vi "Position Error Dialog.vi"(10 "Err Dialog Ref":refnum<vi>, 11 "DAQMan Ref":refnum<vi>) -> (2 "Dialog Ref Out":refnum<vi>)   [LabVIEW 2012, in "Configuration Grandmaster.lvlib" / "FP Controls.lvclass"]
uses:
  FP Controls.lvclass
  <vilib>/Utility/miscctls.llb/LVRectTypeDef.ctl
panel:
  out "output cluster":T1
  out "Front Panel Window:Window Bounds":T1
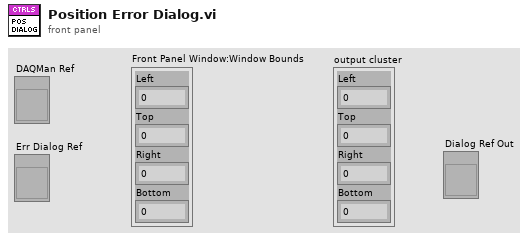
[diagram p1: front panel]
types:
  T1 = typedef "LVRectTypeDef.ctl" = cluster{"Left":i16, "Top":i16, "Right":i16, "Bottom":i16}
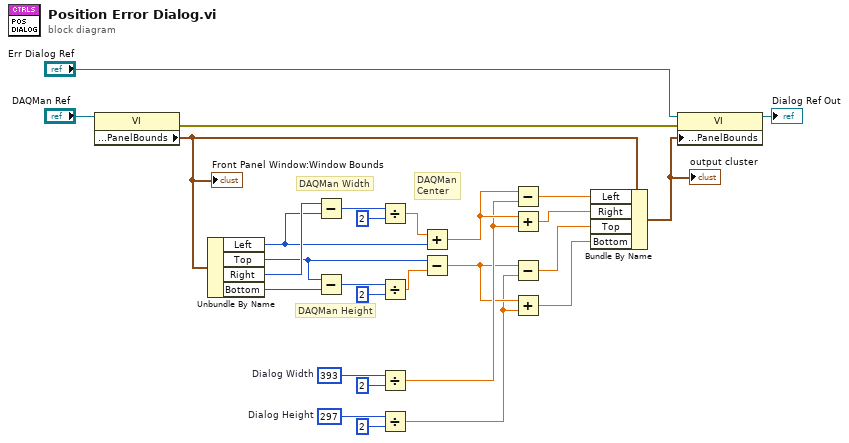
[diagram p0: block diagram]
diagram:
  w16 = i16 297  # Dialog Height
  w18 = i16 393  # Dialog Width
  # "DAQMan\nCenter"
  # "DAQMan Height"
  # "DAQMan Width"
  n1 = property class="VI"(reference="DAQMan Ref") -> (error out=w28:errorcluster, "Front Panel.PanelBounds"=w11:T1)  [unwired: 1 in, 1 out]
  "Front Panel Window:Window Bounds" <- w11
  n2 = Unbundle By Name(w11) -> ("Left"=w15:i16, "Top"=w13:i16, "Right"=w25:i16, "Bottom"=w24:i16)
  n3 = Subtract(x=w25, y=w15) -> (x-y=w23:i16)
  n4 = Subtract(x=w13, y=w24) -> (x-y=w21:i16)
  n5 = Divide(x=w23, y=i16 2) -> (x/y=w14:dbl)
  n6 = Divide(x=w21, y=i16 2) -> (x/y=w12:dbl)
  n7 = Divide(x=w18, y=i16 2) -> (x/y=w8:dbl)
  n8 = Divide(x=w16, y=i16 2) -> (x/y=w4:dbl)
  n9 = Add(x=w14, y=w15) -> (x+y=w9:dbl)
  n10 = Subtract(x=w13, y=w12) -> (x-y=w5:dbl)
  n11 = Subtract(x=w9, y=w8) -> (x-y=w10:dbl)
  n12 = Add(x=w9, y=w8) -> (x+y=w7:dbl)
  n13 = Subtract(x=w5, y=w4) -> (x-y=w6:dbl)
  n14 = Add(x=w5, y=w4) -> (x+y=w3:dbl)
  n15 = Bundle By Name(cluster=w11, "Left"=w10, "Right"=w7, "Top"=w6, "Bottom"=w3) -> (w2:T1)
  "output cluster" <- w2
  n16 = property class="VI"(reference="Err Dialog Ref", error in=w28, "Front Panel.PanelBounds"=w2) -> (reference out=→"Dialog Ref Out":refnum<vi>)  [unwired: 1 out]
